vi "spotkoordinaten.vi"(5 "Gauss":bool, 6 "Area":i32, 7 "Image":dbl[][](array[numeric]), 8 "Particle Reports (Pixels)":T1(array[cluster]), 9 "Center of Mass":cluster{"X":dbl, "Y":dbl}={"X"=-1000.0, "Y"=-1000.0}) -> (0 "Fitted Coefficients":dbl[](array[numeric])=[12.849354442227447, 5.866421178332907, 12.080788064739096, 5.80910915007397, 1224.8335576996235, 9.529730177350924] format="%.2f", 1 "yValues":dbl[](array[numeric]), 2 "Spots":i32, 3 "coefficients of all spots":dbl[][](array[numeric]), 4 "xValues":dbl[](array[numeric]) format="%#_8g")   [LabVIEW 2009]
uses:
  <vilib>/Analysis/NI_AALBase.lvlib
panel:
  in  "LuckyThreshold":dbl=10000.0
  out "Original":dbl[][](graph)
  out "Best Fit":dbl[][](graph)
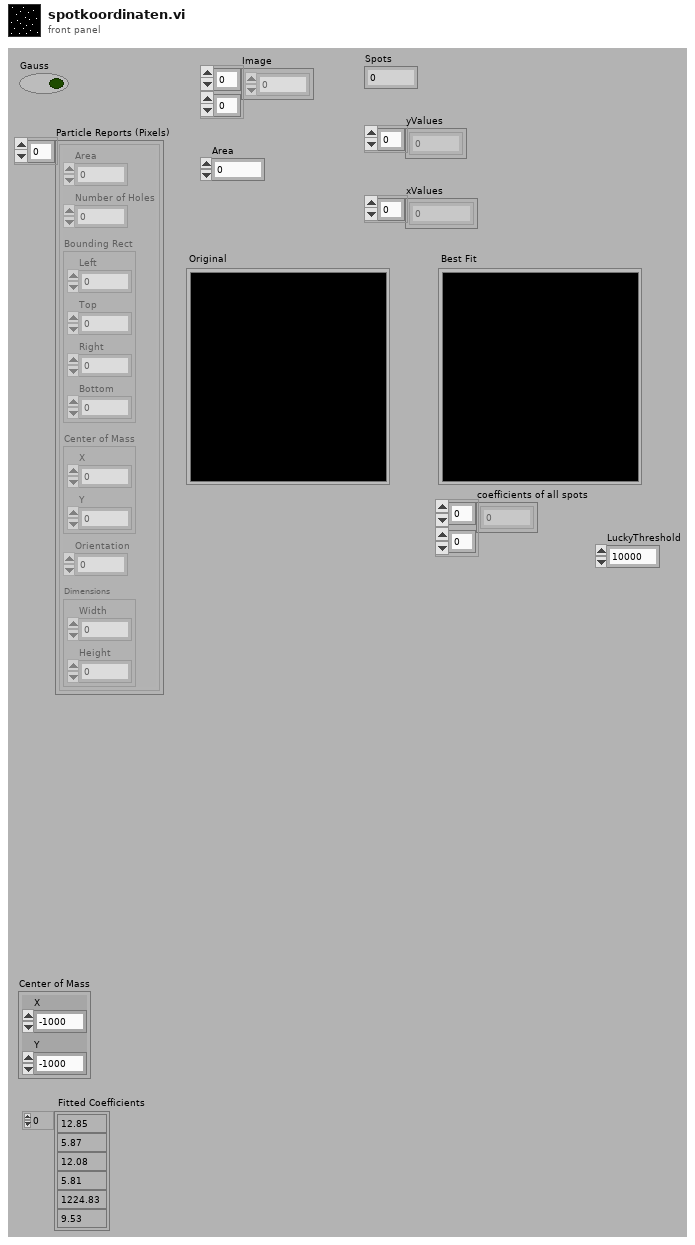
[diagram p1: front panel]
types:
  T1 = cluster{"Area":dbl, "Number of Holes":dbl, "Bounding Rect":cluster{"Left":dbl, "Top":dbl, "Right":dbl, "Bottom":dbl}, "Center of Mass":cluster{"X":dbl, "Y":dbl}, "Orientation":dbl, "Dimensions":cluster{"Width":dbl, "Height":dbl}}[]
  T2 = cluster{"Area":dbl, "Number of Holes":dbl, "Bounding Rect":cluster{"Left":dbl, "Top":dbl, "Right":dbl, "Bottom":dbl}, "Center of Mass":cluster{"X":dbl, "Y":dbl}, "Orientation":dbl, "Dimensions":cluster{"Width":dbl, "Height":dbl}}
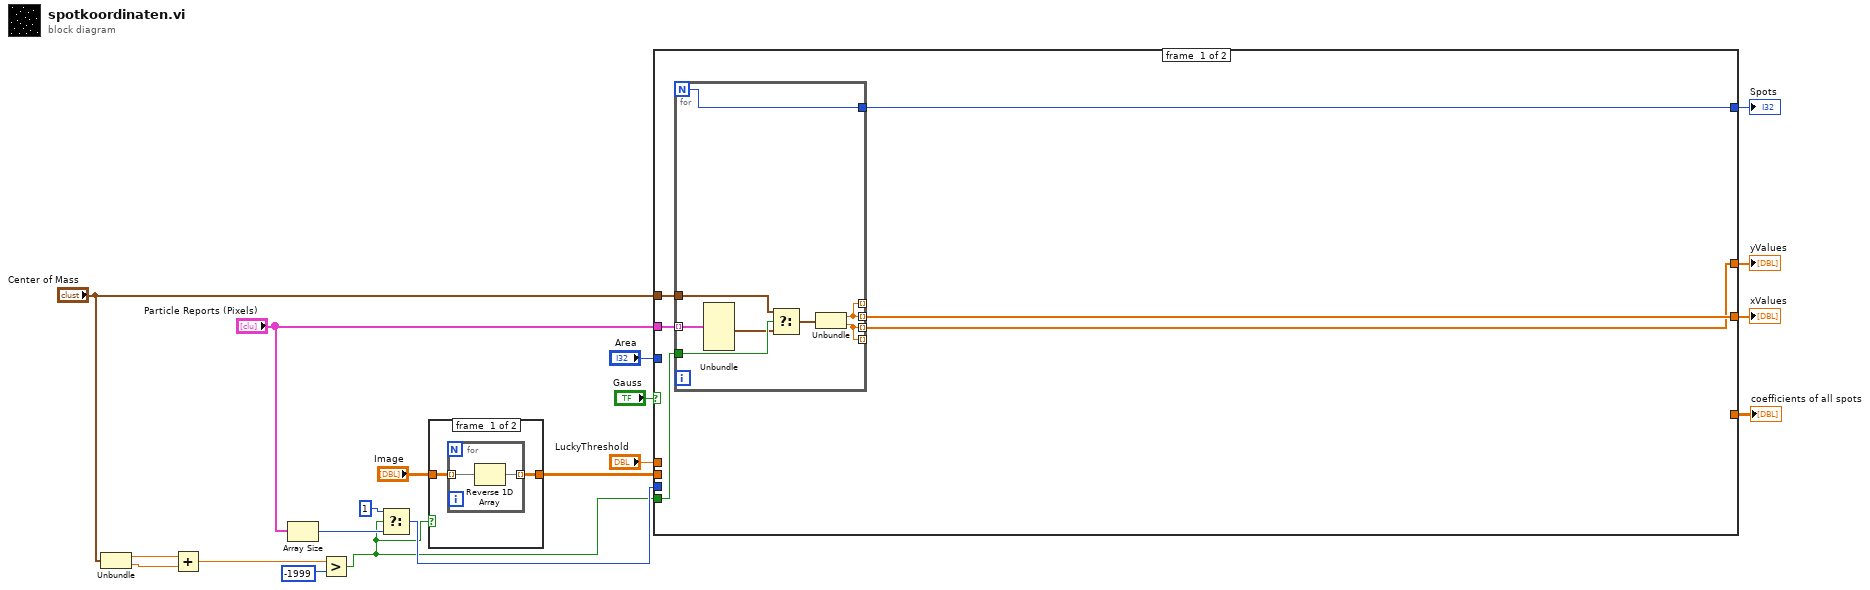
[diagram p0: block diagram]
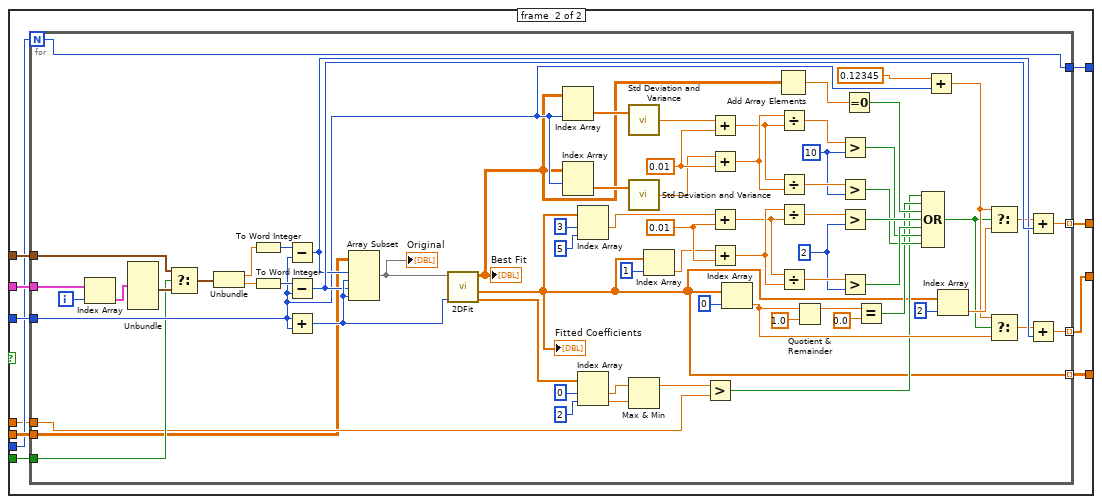
[diagram p3: hidden frame]
diagram:
  n1 = Unbundle("Center of Mass") -> ("X"=w11:dbl, "Y"=w10:dbl)
  n2 = Add(x=w11, y=w10) -> (x+y=w9:dbl)
  n3 = Array Size(array="Particle Reports (Pixels)") -> (size(s)=w5:i32)
  n4 = Greater?(x=w9, y=-1999) -> (0:w3:bool)
  n5 = Select(t=1, s=w3, f=w5) -> (s? t:f=w4:i32)
  n6 = case shown="False" w3 {
    tunnel: "Image" -> [w21 w24]
    tunnel: [w20 w24] -> w14
    frame #0 {
      n7 = for {
        tunnel: w21 -> [w23] mode=indexing
        tunnel: [w22] -> w20 mode=indexing
        n8 = Reverse 1D Array(array=w23) -> (reversed array=w22:dbl[])
      }
    }
    frame #1 {
    }
  }
  n9 = case shown="True" "Gauss" {
    tunnel: [w29 w49] -> w18
    tunnel: [w28 w48] -> w19
    tunnel: "Particle Reports (Pixels)" -> [w30 w47]
    tunnel: w14 -> [_ w46]
    tunnel: "Area" -> [_ w45]
    tunnel: [w27 w44] -> w17
    tunnel: "Center of Mass" -> [w25 w43]
    tunnel: w3 -> [w26 w42]
    tunnel: w4 -> [_ w41]
    tunnel: "LuckyThreshold" -> [_ w40]
    tunnel: [_ w39] -> w1
    frame #0 {
      n10 = for {
        N -> [w37]
        tunnel: w30 -> [w38] mode=indexing
        tunnel: [w36] -> w29 mode=indexing
        tunnel: [w35] -> w28 mode=indexing
        tunnel: [w37] -> w27
        tunnel: [w36] -> _ mode=indexing
        tunnel: [w35] -> _ mode=indexing
        tunnel: w26 -> [w34]
        tunnel: w25 -> [w33]
        n11 = Unbundle(w38) -> ("Center of Mass"=w32:cluster{"X":dbl, "Y":dbl})  [unwired: 5 out]
        n12 = Select(t=w33, s=w34, f=w32) -> (s? t:f=w31:cluster{"X":dbl, "Y":dbl})
        n13 = Unbundle(w31) -> ("X"=w36:dbl, "Y"=w35:dbl)
      }
    }
    frame #1 {
      n14 = for {
        N: w41 -> [w115]
        tunnel: w47 -> [w63]
        tunnel: [w117] -> w49 mode=indexing
        tunnel: [w116] -> w48 mode=indexing
        tunnel: w46 -> [w50]
        tunnel: w45 -> [w102]
        tunnel: [w115] -> w44
        tunnel: w43 -> [w70]
        tunnel: w42 -> [w67]
        tunnel: w40 -> [w54]
        tunnel: [w52] -> w39 mode=indexing
        i -> [w62]
        w85 = 10
        w90 = 0.01
        w94 = 2
        w99 = 0.01
        n15 = Index Array(array=w63, index=w62) -> (element=w61:T2)
        n16 = Unbundle(w61) -> ("Center of Mass"=w69:cluster{"X":dbl, "Y":dbl})  [unwired: 5 out]
        n17 = Select(t=w70, s=w67, f=w69) -> (s? t:f=w68:cluster{"X":dbl, "Y":dbl})
        n18 = Unbundle(w68) -> ("X"=w105:dbl, "Y"=w107:dbl)
        n19 = To Word Integer(number=w105) -> (16bit integer=w106:i16)
        n20 = To Word Integer(number=w107) -> (16bit integer=w108:i16)
        n21 = Subtract(x=w106, y=w102) -> (x-y=w113:i32)
        n22 = Subtract(x=w108, y=w102) -> (x-y=w114:i32)
        n23 = Add(x=w102, y=w102) -> (x+y=w119:i32)
        n24 = Array Subset(array=w50, index (row)=w113, length (row)=w119, index (col)=w114, length (col)=w119) -> (w51:dbl[][])
        "Original" <- w51
        n25 = call "2DFit.vi"("Width Estimate"=w119, "Input image"=w51) -> ("Fitted Errors of Coefficients"=w60:dbl[], "Fitted Coefficients"=w52:dbl[], "Best Fit"=w65:dbl[][])  [unwired: 6 in, 1 out]
        "Best Fit" <- w65
        "Fitted Coefficients" <- w52
        n26 = Index Array(array=w65, index (col)=w102) -> (element=w100:dbl[])  [unwired: 1 in]
        n27 = Index Array(array=w65, index (row)=w102) -> (element=w101:dbl[])  [unwired: 1 in]
        n28 = Index Array(array=w52, index #1=3, index #2=5) -> (element #1=w64:dbl)  [unwired: 1 out]
        n29 = Index Array(array=w60, index #1=0, index #2=2) -> (element #1=w57:dbl, element #2=w56:dbl)
        n30 = call <vilib>:"Std Deviation and Variance.vi"("X"=w100) -> ("standard deviation"=w84:dbl)  [unwired: 1 in, 2 out]
        n31 = call <vilib>:"Std Deviation and Variance.vi"("X"=w101) -> ("standard deviation"=w83:dbl)  [unwired: 1 in, 2 out]
        n32 = Max & Min(x=w57, y=w56) -> (max(x,y)=w55:dbl)  [unwired: 1 out]
        n33 = Index Array(array=w52, index=1) -> (element=w91:dbl)
        n34 = Greater?(x=w55, y=w54) -> (0:w53:bool)
        n35 = Add(x=w84, y=w90) -> (x+y=w88:dbl)
        n36 = Add(x=w83, y=w90) -> (x+y=w89:dbl)
        n37 = Add(x=w64, y=w99) -> (x+y=w97:dbl)
        n38 = Add(x=w91, y=w99) -> (x+y=w98:dbl)
        n39 = Index Array(array=w52, index=0 ("Index")) -> (element=w77:dbl)
        n40 = Add Array Elements(numeric array=w65) -> (sum=w104:dbl)
        n41 = Divide(x=w89, y=w88) -> (x/y=w87:dbl)
        n42 = Divide(x=w88, y=w89) -> (x/y=w86:dbl)
        n43 = Divide(x=w98, y=w97) -> (x/y=w96:dbl)
        n44 = Divide(x=w97, y=w98) -> (x/y=w95:dbl)
        n45 = Quotient & Remainder(x=w77, y=1.0) -> (x-y*floor(x/y)=w74:dbl)  [unwired: 1 out]
        n46 = Greater?(x=w87, y=w85) -> (0:w79:bool)
        n47 = Greater?(x=w86, y=w85) -> (0:w78:bool)
        n48 = Greater?(x=w96, y=w94) -> (0:w81:bool)
        n49 = Greater?(x=w95, y=w94) -> (0:w80:bool)
        n50 = Equal To 0?(x=w104) -> (x = 0?=w82:bool)
        n51 = Equal?(x=w74, y=0.0) -> (x = y?=w73:bool)
        n52 = Compound Arithmetic op=OR(w53, w73, w82, w81, w80, w79, w78) -> (w71:bool)
        n53 = Add(x=0.12345, y=w102) -> (x+y=w109:dbl)
        n54 = Index Array(array=w52, index=2 ("Index")) -> (element=w112:dbl)
        n55 = Select(t=w109, s=w71, f=w112) -> (s? t:f=w110:dbl)
        n56 = Select(t=w109, s=w71, f=w77) -> (s? t:f=w111:dbl)
        n57 = Add(x=w110, y=w114) -> (x+y=w116:dbl)
        n58 = Add(x=w111, y=w113) -> (x+y=w117:dbl)
      }
    }
  }
  "Spots" <- w17
  "yValues" <- w19
  "xValues" <- w18
  "coefficients of all spots" <- w1
